vi "Modbus Convert Temperature.vi"(7 "Divide by 100?":bool, 8 "error in":errorcluster, 11 "PLC Value":i16) -> (0 "error out":errorcluster, 3 "Converted Value":dbl)   [LabVIEW 2023, in "Modbus.lvlib"]
uses:
  Modbus.lvlib
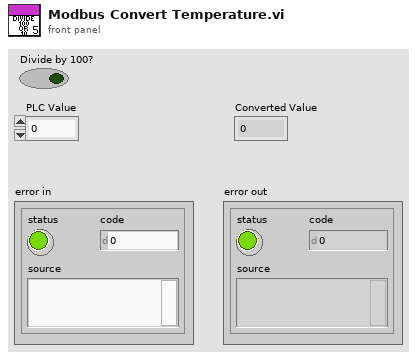
[diagram p1: front panel]
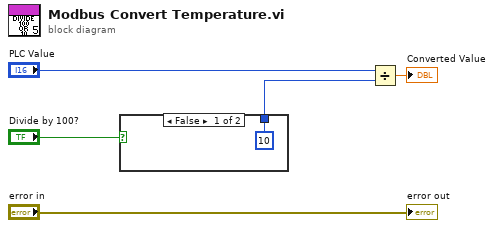
[diagram p0: block diagram]
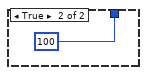
[diagram p2: hidden frame]
diagram:
  n1 = case shown="False" "Divide by 100?" {
    tunnel: [u16 10 ("y") u16 100 ("y")] -> w2
    frame False {
    }
    frame True {
    }
  }
  n2 = Divide(x="PLC Value", y=w2) -> (x/y=→"Converted Value":dbl)
  "error out" <- "error in"
